vi "BufferComicNameNumber.vi"(11 "string in":string) -> (3 "buffered number string":string)   [LabVIEW 2024]
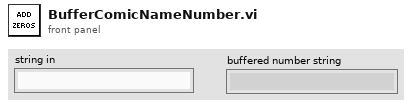
[diagram p1: front panel]
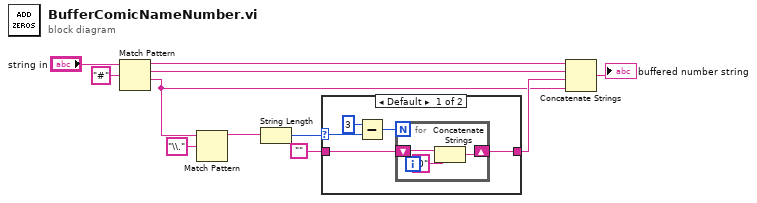
[diagram p0: block diagram]
diagram:
  n1 = Match Pattern(string="string in", regular expression="#") -> (before substring=w9:string, match substring=w8:string, after substring=w3:string)  [unwired: 1 in, 1 out]
  n2 = Match Pattern(string=w3, regular expression="\\.") -> (before substring=w1:string)  [unwired: 1 in, 3 out]
  n3 = String Length(string=w1) -> (length=w10:i32)
  n4 = case shown="Default" w10 {
    selector: w10 -> [w16 _]
    tunnel: [w13 w20] -> w7
    tunnel: "" -> [w12 w20]
    frame Default {
      n5 = Subtract(x=3, y=w16) -> (x-y=w14:i32)
      n6 = for {
        N: w14 -> [_]
        shift-right: [w19] -> w13
        shift-left: w12 -> [w18]
        n7 = Concatenate Strings(w18, "0" ("string")) -> (w19:string)
      }
    }
    frame 3.. {
    }
  }
  n8 = Concatenate Strings(w9, w8, w7, w3) -> (→"buffered number string":string)
